vi "Auto Check Each Tube.vi"(5 "Individual Tube Current In":dbl[](array[numeric]), 6 "error in (no error)":errorcluster, 7 "Failed Tubes In":string[](array[string]), 8 "BoardHandle in":T1, 9 "Barcodes in":string[](array[string]), 10 "Tube #":i32, 11 "Channel # in":i32) -> (0 "BoardHandle out":T1, 1 "error out":errorcluster, 2 "Failed Tubes":string[](array[string]), 3 "Actual Voltage Level (V) 2":dbl format="%#_13g", 4 "Individual Tube Current (Nano Amps)":dbl[](array[numeric]))   [LabVIEW 2020]
uses:
  <instrlib>/CAEN PSM/CAEN PSM.lvlib
panel:
  in  "Individual Tube Current In 4":dbl[](array[numeric])
  out "Individual Tube Current (Nano Amps) 4":dbl[](array[numeric])
  out "error out 4":errorcluster
  out "BoardHandle out 4":T1
  out "Recorded Current\nfor Previous Tube 4":dbl format="%#_13g"
  out "Actual Voltage Level (V) 5":dbl format="%#_13g"
  in  "Individual Tube Current In 3":dbl[](array[numeric])
  out "Individual Tube Current (Nano Amps) 3":dbl[](array[numeric])
  out "error out 3":errorcluster
  out "BoardHandle out 3":T1
  out "Recorded Current\nfor Previous Tube 3":dbl format="%#_13g"
  out "Actual Voltage Level (V) 4":dbl format="%#_13g"
  in  "Individual Tube Current In 2":dbl[](array[numeric])
  out "Individual Tube Current (Nano Amps) 2":dbl[](array[numeric])
  out "error out 2":errorcluster
  out "BoardHandle out 2":T1
  out "Recorded Current\nfor Previous Tube 2":dbl format="%#_13g"
  out "Actual Voltage Level (V) 3":dbl format="%#_13g"
  out "Recorded Current\nfor Previous Tube":dbl format="%#_13g"
  out "Next Measurment":string
  # "future developement"
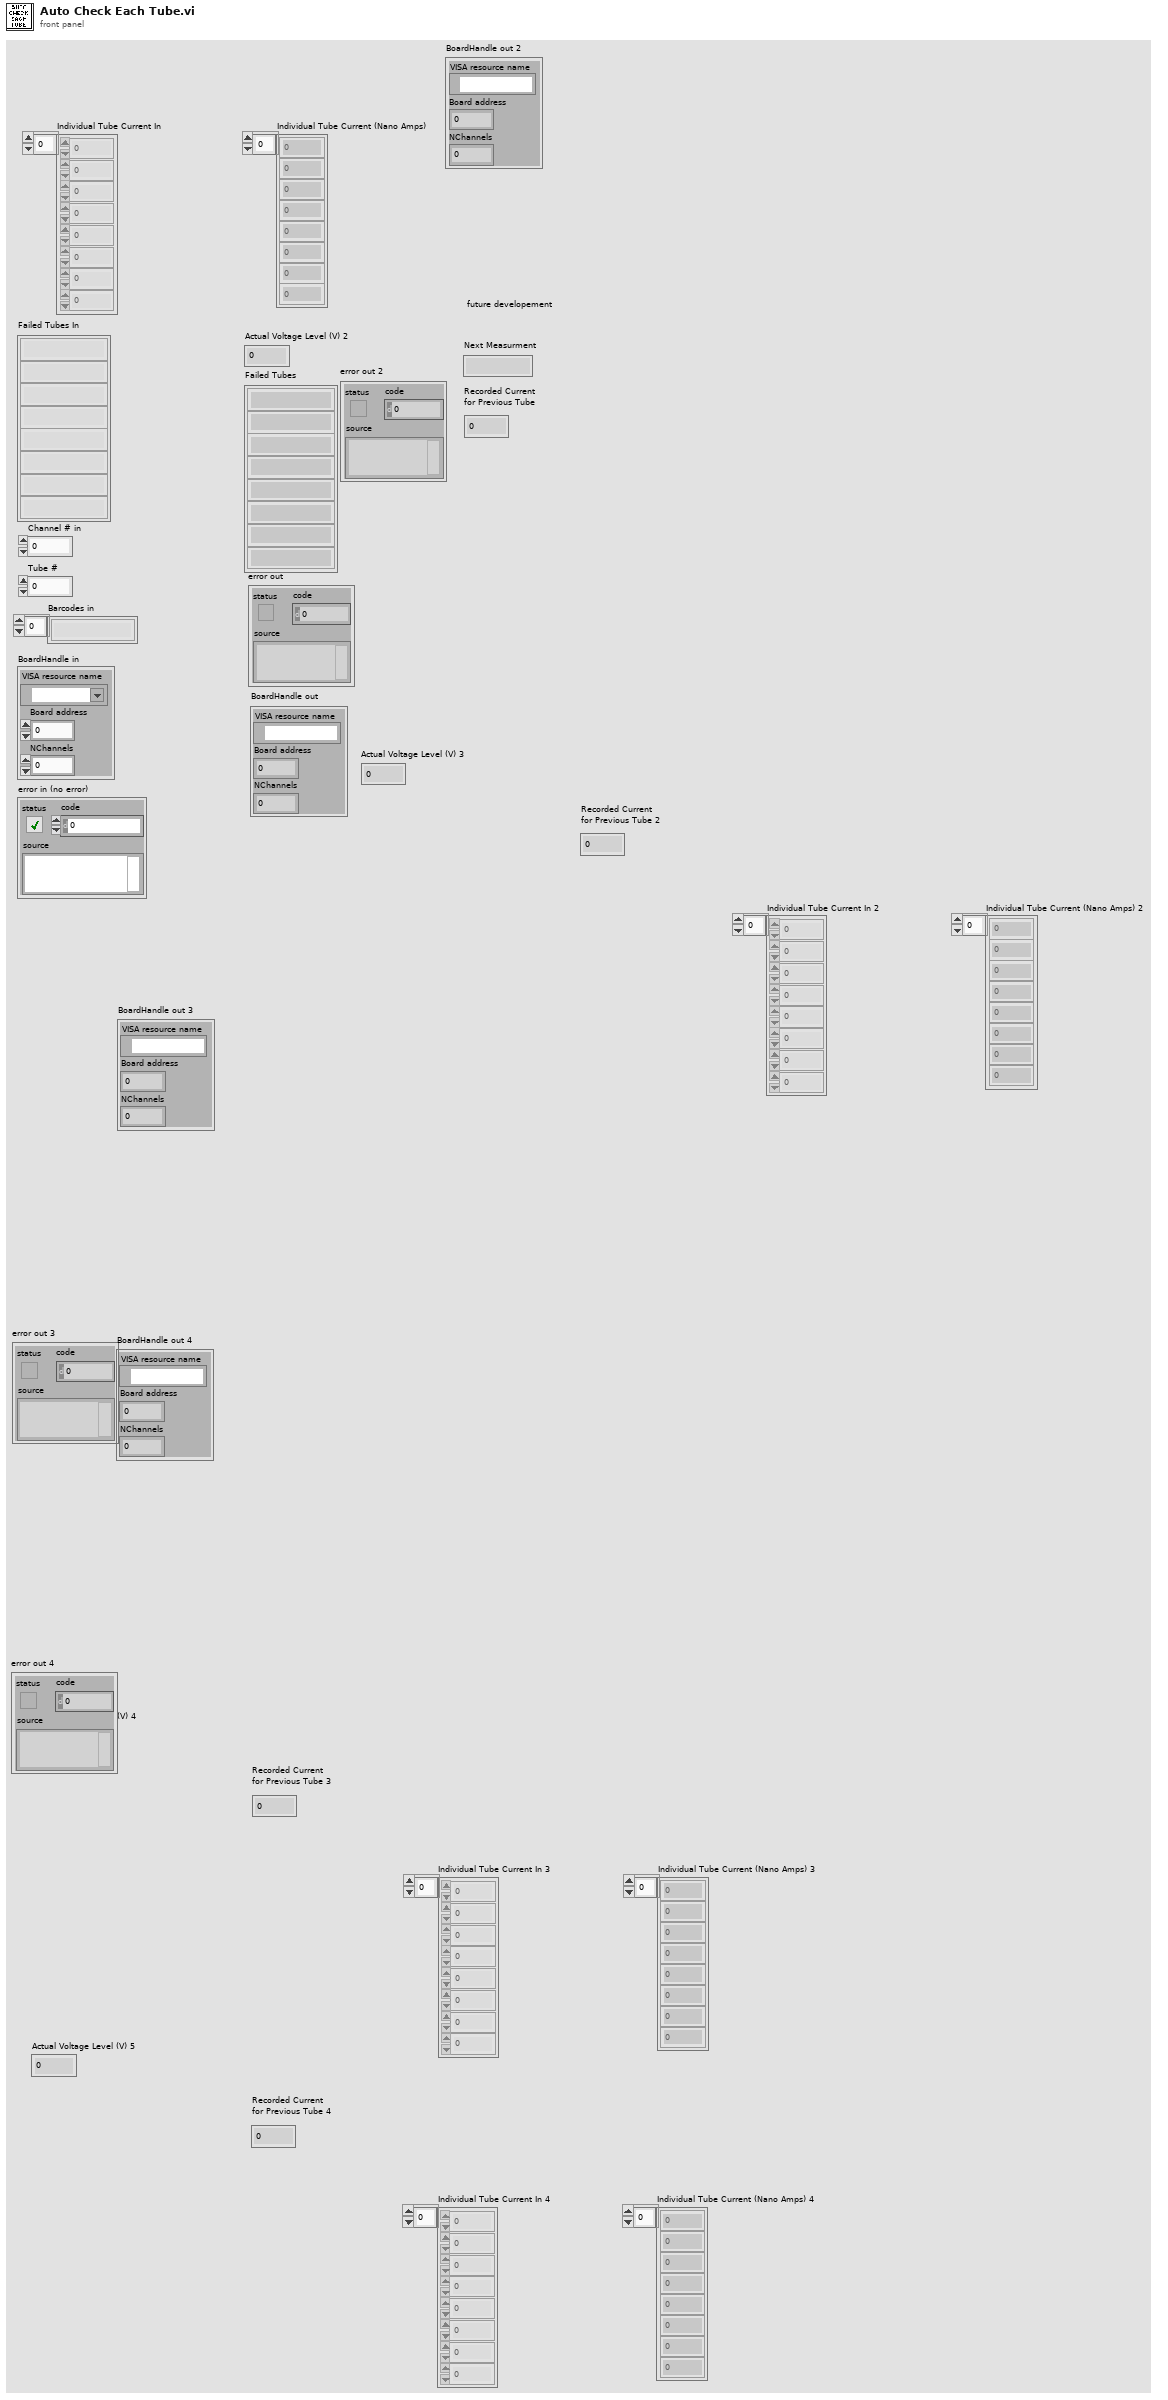
[diagram p1: front panel]
types:
  T1 = cluster{"VISA resource name":refnum<visa-resource-name>, "Board address":u8, "NChannels":u8}
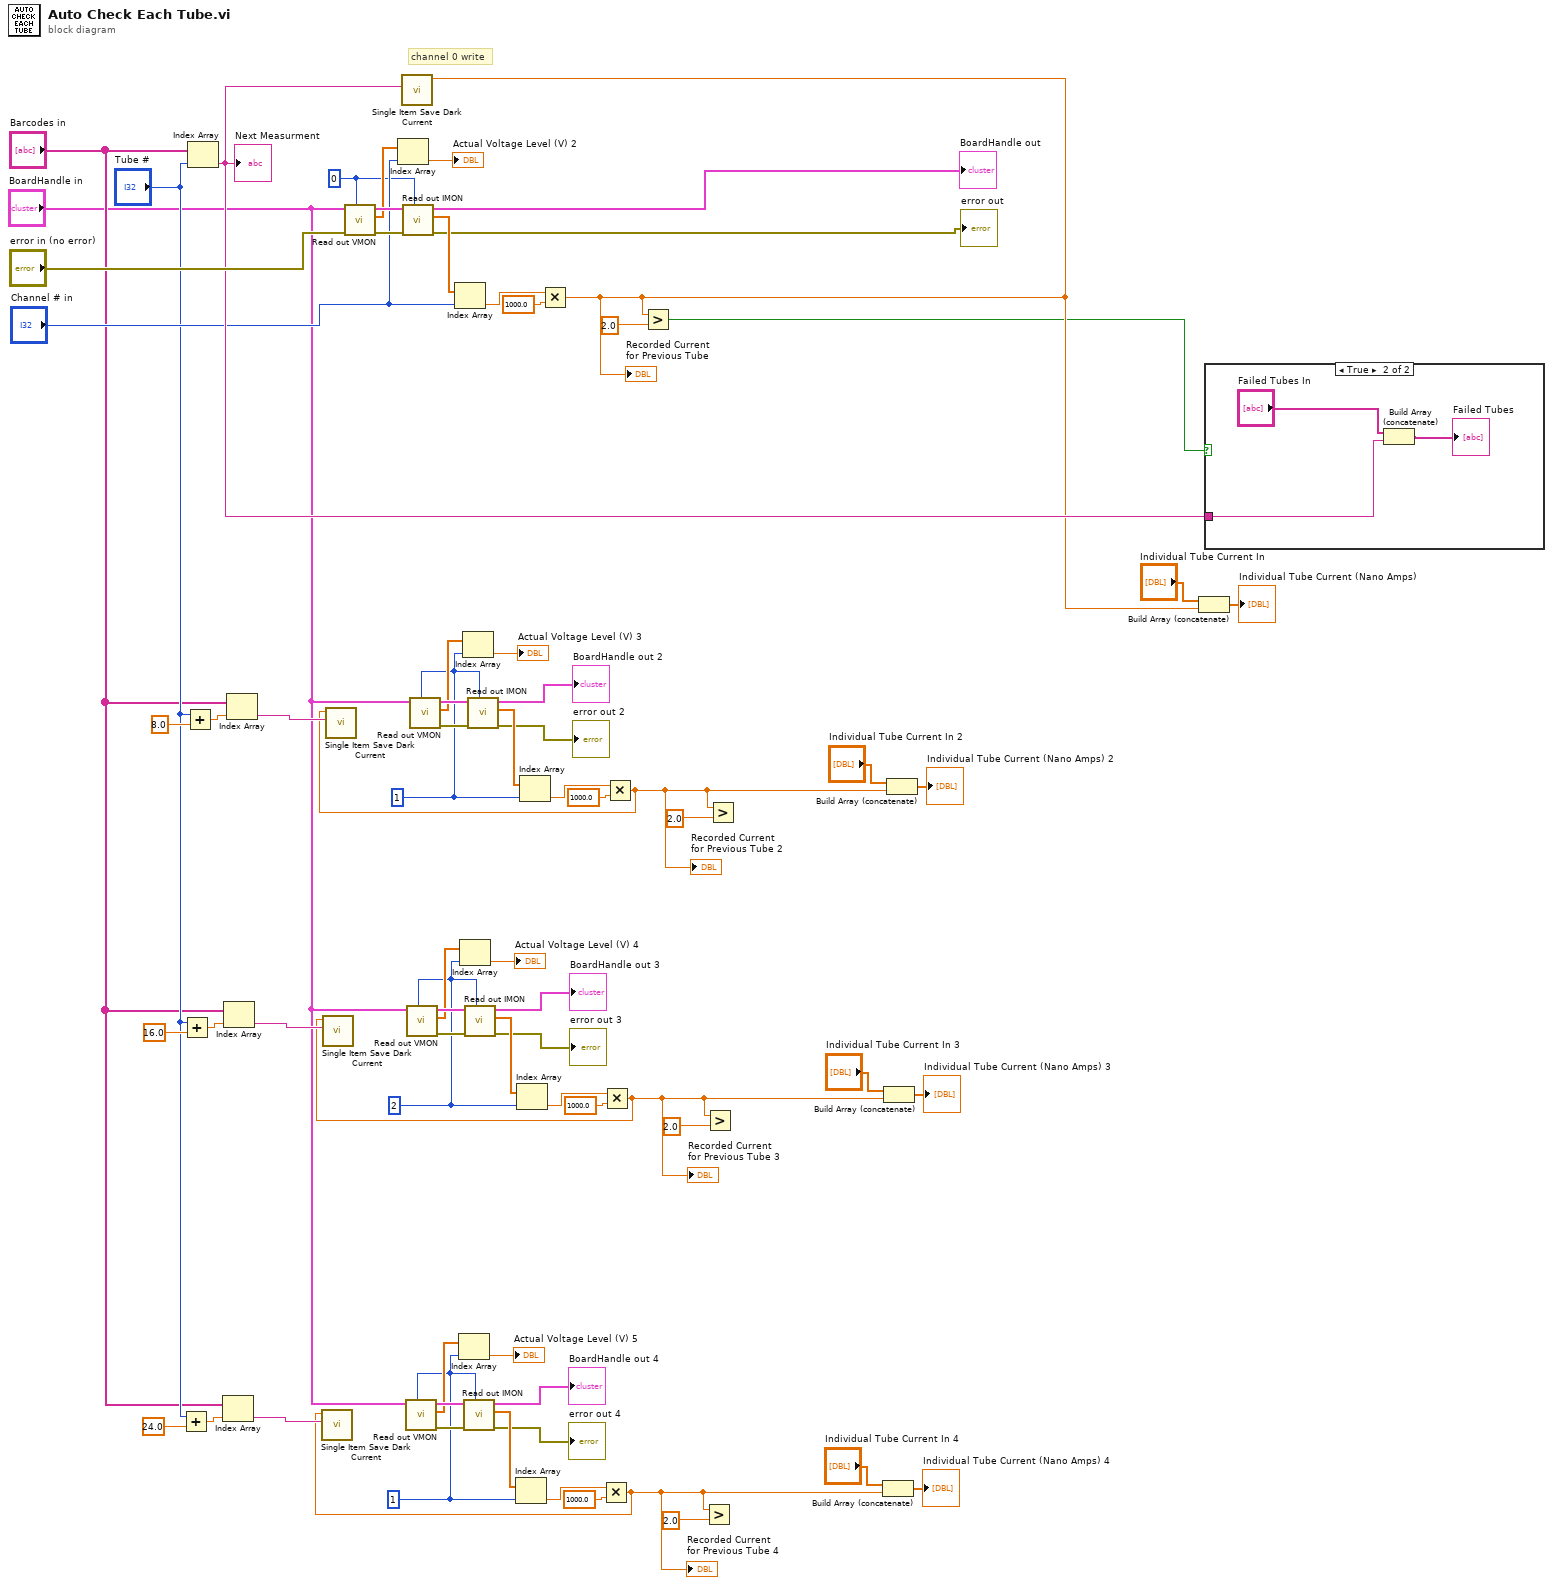
[diagram p0: block diagram]
diagram:
  w12 = 1 ("index")
  w29 = 2 ("index")
  w49 = 1 ("index")
  w58 = u8 0 ("Channel")
  # "channel 0 write"
  n1 = Add(x="Tube #", y=24.0) -> (x+y=w11:dbl)
  n2 = Add(x="Tube #", y=16.0) -> (x+y=w28:dbl)
  n3 = Add(x="Tube #", y=8.0) -> (x+y=w48:dbl)
  n4 = Index Array(array="Barcodes in", index="Tube #") -> (element=w63:string)
  "Next Measurment" <- w63
  n5 = Index Array(array="Barcodes in", index=w11) -> (element=w9:string)
  n6 = Index Array(array="Barcodes in", index=w28) -> (element=w26:string)
  n7 = Index Array(array="Barcodes in", index=w48) -> (element=w45:string)
  n8 = call <instrlib>:"Read out VMON.vi"("Channel"=w58, "error in (no error)"="error in (no error)", "BoardHandle"="BoardHandle in") -> ("error out"=w67:errorcluster, "VMon values (V)"=w65:dbl[], "BoardHandle out"=w66:T1)  [unwired: 6 in]
  n9 = Index Array(array=w65, index="Channel # in") -> (element=→"Actual Voltage Level (V) 2":dbl)
  n10 = call <instrlib>:"Read out IMON.vi"("Channel"=w58, "error in (no error)"=w67, "BoardHandle"=w66) -> ("error out"=→"error out":errorcluster, "IMon values (uA)"=w70:dbl[], "BoardHandle out"=→"BoardHandle out":T1)  [unwired: 5 in, 1 out]
  n11 = call <instrlib>:"Read out VMON.vi"("Channel"=w12, "BoardHandle"="BoardHandle in") -> ("error out"=w16:errorcluster, "VMon values (V)"=w14:dbl[], "BoardHandle out"=w15:T1)  [unwired: 7 in]
  n12 = call <instrlib>:"Read out VMON.vi"("Channel"=w29, "BoardHandle"="BoardHandle in") -> ("error out"=w33:errorcluster, "VMon values (V)"=w31:dbl[], "BoardHandle out"=w32:T1)  [unwired: 7 in]
  n13 = call <instrlib>:"Read out VMON.vi"("Channel"=w49, "BoardHandle"="BoardHandle in") -> ("error out"=w53:errorcluster, "VMon values (V)"=w51:dbl[], "BoardHandle out"=w52:T1)  [unwired: 7 in]
  n14 = Index Array(array=w70, index="Channel # in") -> (element=w68:dbl)
  n15 = Index Array(array=w14, index=w12) -> (element=→"Actual Voltage Level (V) 5":dbl)
  n16 = Index Array(array=w31, index=w29) -> (element=→"Actual Voltage Level (V) 4":dbl)
  n17 = Index Array(array=w51, index=w49) -> (element=→"Actual Voltage Level (V) 3":dbl)
  n18 = call <instrlib>:"Read out IMON.vi"("Channel"=w12, "error in (no error)"=w16, "BoardHandle"=w15) -> ("error out"=→"error out 4":errorcluster, "IMon values (uA)"=w19:dbl[], "BoardHandle out"=→"BoardHandle out 4":T1)  [unwired: 5 in, 1 out]
  n19 = call <instrlib>:"Read out IMON.vi"("Channel"=w29, "error in (no error)"=w33, "BoardHandle"=w32) -> ("error out"=→"error out 3":errorcluster, "IMon values (uA)"=w36:dbl[], "BoardHandle out"=→"BoardHandle out 3":T1)  [unwired: 5 in, 1 out]
  n20 = call <instrlib>:"Read out IMON.vi"("Channel"=w49, "error in (no error)"=w53, "BoardHandle"=w52) -> ("error out"=→"error out 2":errorcluster, "IMon values (uA)"=w56:dbl[], "BoardHandle out"=→"BoardHandle out 2":T1)  [unwired: 5 in, 1 out]
  n21 = Index Array(array=w19, index=w12) -> (element=w17:dbl)
  n22 = Index Array(array=w36, index=w29) -> (element=w34:dbl)
  n23 = Index Array(array=w56, index=w49) -> (element=w54:dbl)
  n24 = Multiply(x=w68, y=1000.0) -> (x*y=w62:dbl)
  "Recorded Current\nfor Previous Tube" <- w62
  n25 = call "Single Item Save Dark Current.vi"("String"=w63, "Numeric"=w62) -> ()  [unwired: 10 in]
  n26 = Multiply(x=w17, y=1000.0) -> (x*y=w4:dbl)
  "Recorded Current\nfor Previous Tube 4" <- w4
  n27 = call "Single Item Save Dark Current.vi"("String"=w9, "Numeric"=w4) -> ()  [unwired: 10 in]
  n28 = Multiply(x=w34, y=1000.0) -> (x*y=w21:dbl)
  "Recorded Current\nfor Previous Tube 3" <- w21
  n29 = call "Single Item Save Dark Current.vi"("String"=w26, "Numeric"=w21) -> ()  [unwired: 10 in]
  n30 = Multiply(x=w54, y=1000.0) -> (x*y=w38:dbl)
  "Recorded Current\nfor Previous Tube 2" <- w38
  n31 = call "Single Item Save Dark Current.vi"("String"=w45, "Numeric"=w38) -> ()  [unwired: 10 in]
  n32 = Greater?(x=w62, y=2.0) -> (0:w46:bool)
  n33 = Greater?(x=w4, y=2.0) -> ()  [unwired: 1 out]
  n34 = Greater?(x=w21, y=2.0) -> ()  [unwired: 1 out]
  n35 = Greater?(x=w38, y=2.0) -> ()  [unwired: 1 out]
  n36 = Build Array (concatenate)("Individual Tube Current In 4", w4) -> (→"Individual Tube Current (Nano Amps) 4":dbl[])
  n37 = Build Array (concatenate)("Individual Tube Current In 3", w21) -> (→"Individual Tube Current (Nano Amps) 3":dbl[])
  n38 = Build Array (concatenate)("Individual Tube Current In 2", w38) -> (→"Individual Tube Current (Nano Amps) 2":dbl[])
  n39 = Build Array (concatenate)("Individual Tube Current In", w62) -> (→"Individual Tube Current (Nano Amps)":dbl[])
  n40 = case shown="True" w46 {
    tunnel: w63 -> [_ w74]
    frame False {
    }
    frame True {
      n41 = Build Array (concatenate)("Failed Tubes In", w74) -> (→"Failed Tubes":string[])
    }
  }
